vi "Read Data From Instrument.vi"(8 "error in (no error)":errorcluster, 10 "File (\"INT:\\ARB_001.arb\")":string="INT:\\ARB_001.arb", 11 "VISA resource name":refnum<visa-resource-name>) -> (0 "error out":errorcluster, 2 "Instrument Data":string, 3 "VISA resource name out":refnum<visa-resource-name>)   [LabVIEW 2020, in "Agilent 3352X Series.lvlib"]
doc: "Reads the contents of a specified file in the instrument."
uses:
  Agilent 3352X Series.lvlib
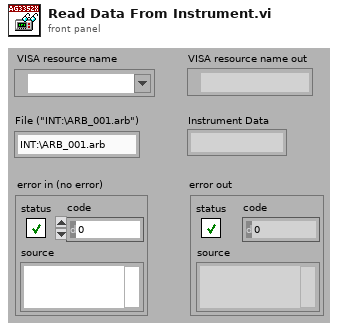
[diagram p1: front panel]
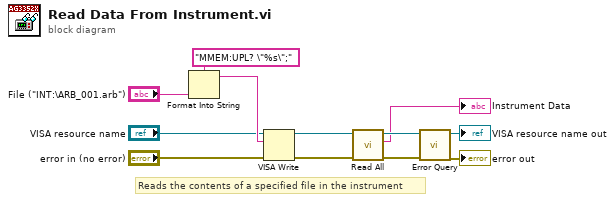
[diagram p0: block diagram]
diagram:
  # "Reads the contents of a specified file in the instrument"
  n1 = Format Into String(format string="MMEM:UPL? \"%s\";", "File (\"INT:\\ARB_001.arb\")") -> (resulting string=w10:string)  [unwired: 2 in, 1 out]
  n2 = VISA Write(VISA resource name="VISA resource name", write buffer=w10, error in (no error)="error in (no error)") -> (VISA resource name out=w5:refnum<visa-resource-name>, error out=w3:errorcluster)  [unwired: 1 out]
  n3 = call "Read All.vi"("error in (no error)"=w3, "VISA resource name"=w5) -> ("error out"=w2:errorcluster, "Data String"=→"Instrument Data":string, "VISA resource name out"=w4:refnum<visa-resource-name>)  [unwired: 7 out]
  n4 = call "Error Query.vi"("error in (no error)"=w2, "VISA resource name"=w4) -> ("error out"=→"error out":errorcluster, "VISA resource name out"=→"VISA resource name out":refnum<visa-resource-name>)  [unwired: 8 out]
